vi "StringTo1DI8.vi"(0 "String":string, 7 "Offset":i32 caption="Offset (0)", 11 "Error in":errorcluster caption="Error in (no error)") -> (4 "Array":i8[](array[numeric]), 8 "Offset Past Array":i32, 15 "Error out":errorcluster)   [LabVIEW 2017, in "GPString.lvlib"]
doc: "Converts <B>String</B> to <B>Array</B>, starting the conversion from the optional <B>Offset</B> in <B>String</B>.\n\n<B>String formatting</B>\n- Element separator character must be \";\".\n- Array enclosure characters can be either square or curly brackets.\n\nThis VI is inlined.\n\nSteen Schmidt\nGPower\n15/6 2016"
uses:
  GPString.lvlib
panel:
  # "Copyright © 2016\nGPower\nSee enclosed license file for terms and conditions"
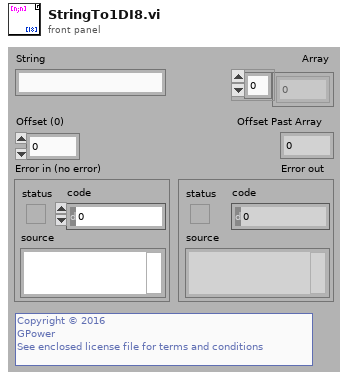
[diagram p1: front panel]
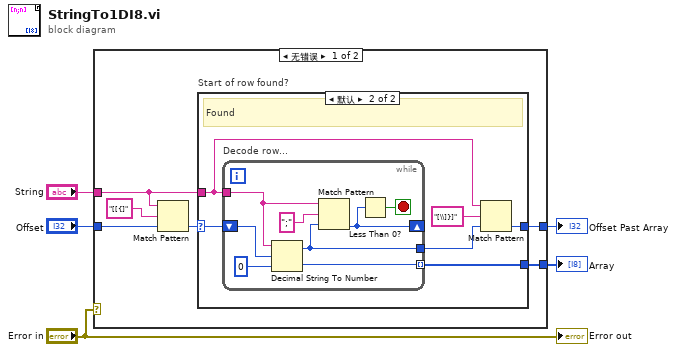
[diagram p0: block diagram]
diagram:
  n1 = case shown="无错误" "Error in" {
    tunnel: "String" -> [w8 _]
    tunnel: "Offset" -> [w6 w27]
    tunnel: [w10 _] -> w3
    tunnel: [w9 w27] -> w2
    frame No Error {
      n2 = Match Pattern(string=w8, regular expression="[[{]", offset (0)=w6) -> (offset past match=w7:i32)  [unwired: 3 out]
      n3 = case "Start of row found?" shown="默认" w7 {
        selector: w7 -> [w12 w13]
        tunnel: [_ w18] -> w10
        tunnel: [w12 w16] -> w9
        tunnel: w8 -> [_ w14]
        frame -1 {
          # "Not found"
        }
        frame Default {
          # "Found"
          n4 = while "Decode row..." {
            tunnel: w14 -> [w25]
            shift-right: [w23] -> _
            shift-left: w13 -> [w24]
            tunnel: [w20] -> w18 mode=indexing
            tunnel: [w21] -> w15
            stop <- w22 stop-if-true
            n5 = Decimal String To Number(string=w25, offset=w24, default (0L)=i8 0) -> (offset past number=w21:i32, number=w20:i8)
            n6 = Match Pattern(string=w25, regular expression=";", offset (0)=w21) -> (offset past match=w23:i32)  [unwired: 3 out]
            n7 = Less Than 0?(x=w23) -> (x < 0?=w22:bool)
          }
          n8 = Match Pattern(string=w14, regular expression="[\\]}]", offset (0)=w15) -> (offset past match=w16:i32)  [unwired: 3 out]
        }
      }
    }
    frame Error {
    }
  }
  "Array" <- w3
  "Offset Past Array" <- w2
  "Error out" <- "Error in"
